vi "getFlags.vi"(11 "SUBSCRIBE in":refnum<class "SUBSCRIBE.lvclass">) -> (0 "RETAIN":bool, 1 "QoS":T1, 2 "DUP":bool, 3 "SUBSCRIBE out":refnum<class "SUBSCRIBE.lvclass">)   [LabVIEW 2013, in "SUBSCRIBE.lvclass"]
uses:
  SUBSCRIBE.lvclass
  ControlPacket/QualityOfService -- enum.ctl
  ControlPacket/ControlPacket.lvclass
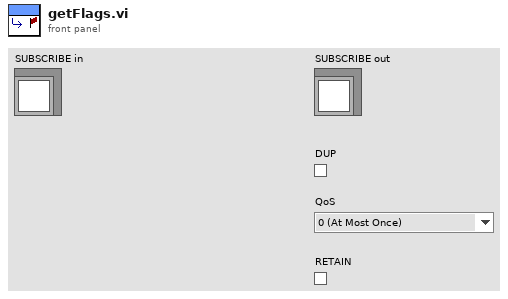
[diagram p1: front panel]
types:
  T1 = typedef "ControlPacket.lvclass/QualityOfService -- enum.ctl" = enum16{"0 (At Most Once)", "1 (At Least Once)", "2 (Exactly Once)"}
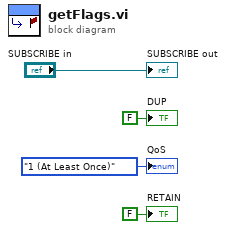
[diagram p0: block diagram]
diagram:
  "SUBSCRIBE out" <- "SUBSCRIBE in"
  "QoS" <- QualityOfService_--_enum."1 (At Least Once)" ("QoS")
  "DUP" <- FALSE ("DUP")
  "RETAIN" <- FALSE ("RETAIN")
